vi "Read IPS120.vi"(8 "error in (no error)":errorcluster, 9 "Divide by":dbl=1.0, 11 "VISA resource name":refnum<visa-resource-name>) -> (0 "error out":errorcluster, 1 "read buffer":string, 2 "Value":dbl, 3 "VISA resource name out":refnum<visa-resource-name>, 4 "Repeats":i32)   [LabVIEW 2019]
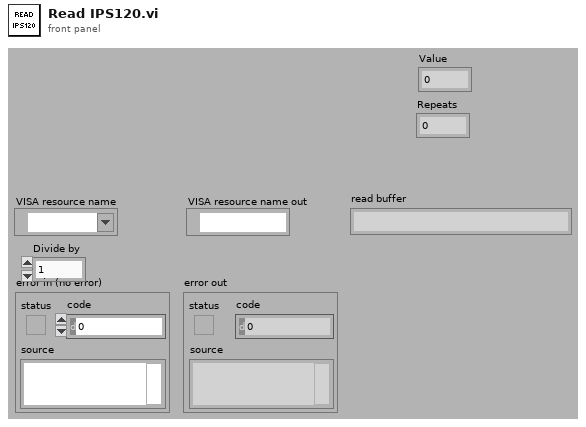
[diagram p1: front panel]
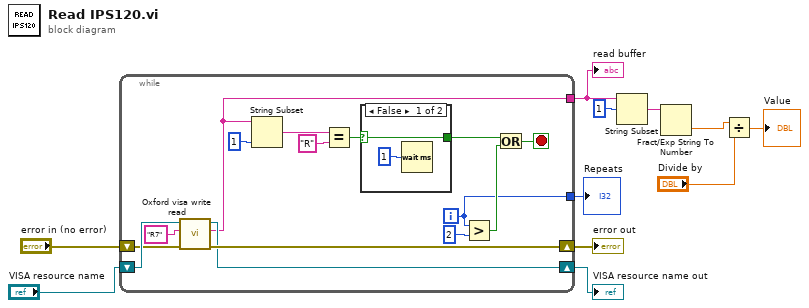
[diagram p0: block diagram]
diagram:
  n1 = while {
    tunnel: [w20] -> w7
    shift-right: [w23] -> w8
    shift-left: "VISA resource name" -> [w26]
    shift-right: [w24] -> w9
    shift-left: "error in (no error)" -> [w25]
    tunnel: [w12] -> w4
    i -> [w12]
    stop <- w14 stop-if-true
    n2 = call "Oxford visa write read.vi"("error in (no error)"=w25, "write buffer"="R7", "VISA resource name"=w26) -> ("error out"=w24:errorcluster, "read buffer"=w20:string, "VISA resource name out"=w23:refnum<visa-resource-name>)  [unwired: 6 in]
    n3 = String Subset(string=w20, length (rest)=1 ("length (rest)")) -> (substring=w19:string)  [unwired: 1 in]
    n4 = Equal?(x=w19, y="R") -> (x = y?=w17:bool)
    n5 = case shown="False" w17 {
      selector: w17 -> [w27 w29]
      tunnel: [w27 w29] -> w16
      frame False {
        n6 = Wait (ms)(milliseconds to wait=u32 1) -> ()  [unwired: 1 out]
      }
      frame True {
      }
    }
    n7 = Greater?(x=w12, y=2) -> (0:w13:bool)
    n8 = Or(x=w16, y=w13) -> (x .or. y?=w14:bool)
  }
  "VISA resource name out" <- w8
  "error out" <- w9
  "read buffer" <- w7
  "Repeats" <- w4
  n9 = String Subset(string=w7, offset (0)=1) -> (substring=w5:string)  [unwired: 1 in]
  n10 = Fract/Exp String To Number(string=w5) -> (number=w2:dbl)  [unwired: 3 in, 1 out]
  n11 = Divide(x=w2, y="Divide by") -> (x/y=→"Value":dbl)
